vi "禹山电导率_获取用户校准参数.vi"(8 "error in (no error)":errorcluster caption="错误输入（无错误）", 11 "MB session in":refnum<class "MB_Master.lvclass">) -> (0 "error out":errorcluster caption="错误输出", 2 "输出值":cluster{"K":sgl, "B":sgl}, 3 "MB session out":refnum<class "MB_Master.lvclass">)   [LabVIEW 2016, in "斯坦道多参数.lvlib"]
uses:
  <vilib>/Plasmionique/MB Master/MB_Master/MB_Master.lvclass
  <vilib>/Plasmionique/MB Master/MB Master.lvlib
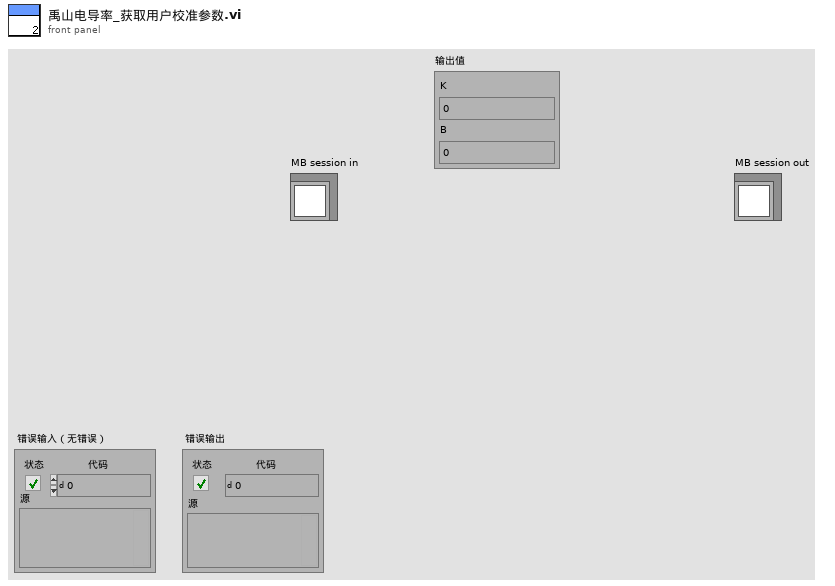
[diagram p1: front panel]
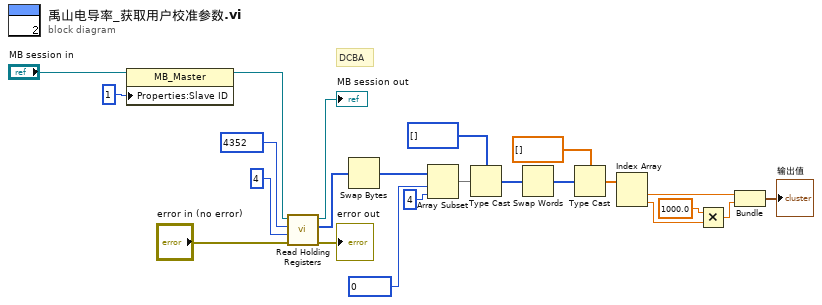
[diagram p0: block diagram]
diagram:
  # "DCBA"
  n1 = property class="MB_Master"(reference="MB session in", "Properties:Slave ID"=u16 1 ("y")) -> (reference out=w11:refnum<class "MB_Master.lvclass">)  [unwired: 1 in, 1 out]
  n2 = call <vilib>:"Read Holding Registers.vi"("error in (no error)"="error in (no error)", "quantity"=u16 4, "starting address"=u16 4352, "MB session in"=w11) -> ("error out"=→"error out":errorcluster, "Registers"=w8:u16[], "MB session out"=→"MB session out":refnum<class "MB_Master.lvclass">)  [unwired: 5 in]
  n3 = Swap Bytes(anything=w8) -> (byte swapped=w7:u16[])
  n4 = Array Subset(array=w7, index=u16 0 ("starting address"), length=4 ("长度")) -> (w6:u16[])
  n5 = Type Cast(type=u32[] [] ("数组 2"), x=w6) -> (*(type *) &x=w18:u32[])
  n6 = Swap Words(1:w18) -> (0:w20:u32[])
  n7 = Type Cast(type=sgl[] [] ("数组 2"), x=w20) -> (*(type *) &x=w16:sgl[])
  n8 = Index Array(array=w16) -> (element #1=w15:sgl, element #2=w14:sgl)  [unwired: 2 in]
  n9 = Multiply(x=sgl 1000.0, y=w14) -> (x*y=w2:sgl)
  n10 = Bundle("数值"=w15, w2) -> (→"输出值":cluster{"数值":sgl, sgl})  [unwired: 1 in]
